vi "CAN Communication.vi"(7 "CAN Mode":T1, 8 "Error IN":errorcluster, 10 "Message":u8[](array[numeric]), 11 "Arbitration ID":u32) -> (0 "Error OUT":errorcluster, 3 "CAN Ref":refnum<k20>)   [LabVIEW 2019]
uses:
  Type Defs/CAN Mode.ctl
  <vilib>/RioEmbeddedCAN/RioEmbeddedCAN.llb/CANFrameControl.ctl
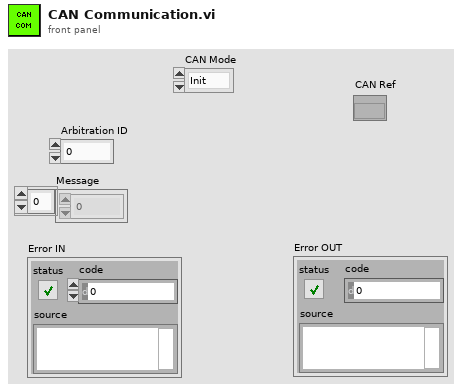
[diagram p1: front panel]
types:
  T1 = typedef "CAN Mode.ctl" = enum16{"Init", "Read", "Write", "Close"}
  T2 = typedef "CANFrameControl.ctl" = cluster{"identifier":u32, "extended?":bool, "type":u8, "payload":u8[]}
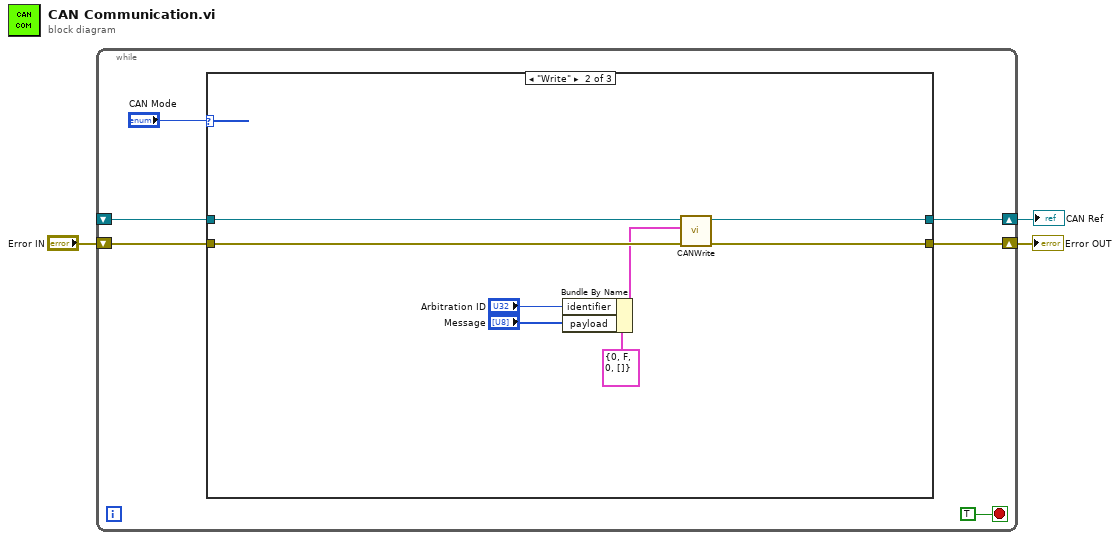
[diagram p0: block diagram]
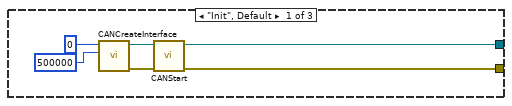
[diagram p2: hidden frame]
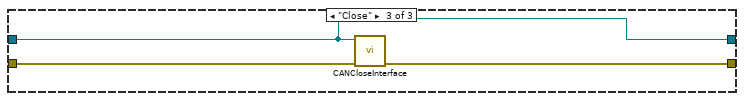
[diagram p3: hidden frame]
diagram:
  n1 = while {
    shift-right: [w7] -> w1
    shift-left: _ -> [w5]
    shift-right: [w6] -> w2
    shift-left: "Error IN" -> [w4]
    stop <- TRUE stop-if-true
    n2 = case shown="\"Write\"" "CAN Mode" {
      tunnel: [w11 w21 w24] -> w7
      tunnel: [w10 w16 w25] -> w6
      tunnel: w5 -> [_ w23 w24]
      tunnel: w4 -> [_ w22 w26]
      frame "Init", Default {
        n3 = call <vilib>:"CANCreateInterface.vi"("baud rate (125000 bps)"=u32 500000 ("baud rate"), "interface index"=u32 0) -> ("error out"=w12:errorcluster, "interface object out"=w13:refnum<k20>)  [unwired: 8 in]
        n4 = call <vilib>:"CANStart.vi"("error in (no error)"=w12, "interface object in"=w13) -> ("error out"=w10:errorcluster, "interface object out"=w11:refnum<k20>)  [unwired: 8 in]
      }
      frame "Write" {
        n5 = Bundle By Name(cluster=T2 {"identifier"=0, "extended?"=FALSE, "type"=0, "payload"=[]} ("CAN frame"), "identifier"="Arbitration ID", "payload"="Message") -> (w19:T2)
        n6 = call <vilib>:"CANWrite.vi"("error in (no error)"=w22, "CAN frame"=w19, "interface object in"=w23) -> ("error out"=w16:errorcluster, "interface object out"=w21:refnum<k20>)  [unwired: 7 in]
      }
      frame "Close" {
        n7 = call <vilib>:"CANCloseInterface.vi"("error in (no error)"=w26, "interface object in"=w24) -> ("error out"=w25:errorcluster)  [unwired: 9 in]
      }
    }
  }
  "Error OUT" <- w2
  "CAN Ref" <- w1
